vi "Find Relay Index.vi"(8 "error in (no error)":errorcluster, 10 "relay string":string, 11 "SLSC Switch in":refnum<class "SLSC Switch.lvclass">) -> (0 "error out":errorcluster, 2 "index":i32, 3 "SLSC Switch out":refnum<class "SLSC Switch.lvclass">)   [LabVIEW 2016, in "SLSC Switch.lvlib" / "SLSC Switch.lvclass"]
uses:
  SLSC Switch.lvclass
  SLSC Switch.lvclass/SLSC Switch.ctl
  Switch Action Processor/Switch Action Processor.lvclass/Switch Action Processor.ctl
  Relay/Relay.lvclass/Relay.ctl
  Relay/Relay.lvclass
  Switch Action Processor/Switch Action Processor.lvclass
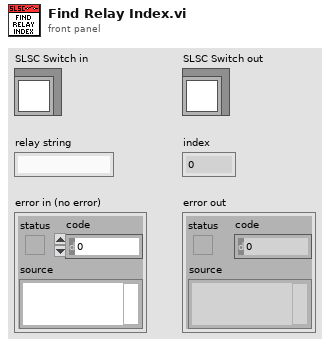
[diagram p1: front panel]
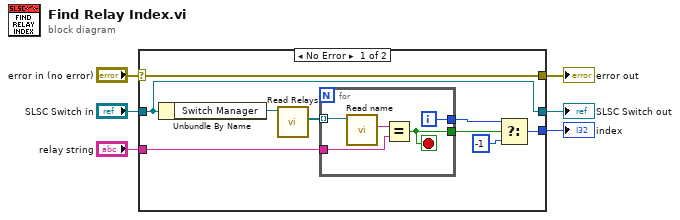
[diagram p0: block diagram]
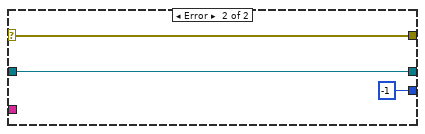
[diagram p2: hidden frame]
diagram:
  n1 = case shown="No Error" "error in (no error)" {
    selector: "error in (no error)" -> [w13 w23]
    tunnel: [w13 w23] -> w5
    tunnel: "relay string" -> [w15 _]
    tunnel: [w14 -1 ("index of element")] -> w3
    tunnel: "SLSC Switch in" -> [w9 w21]
    tunnel: [w9 w21] -> w1
    frame No Error {
      n2 = Unbundle By Name(w9) -> ("Switch Manager"=w8:refnum<class "Switch Action Processor.lvclass">)
      n3 = call "Read Relays.vi"("Switch Action Processor in"=w8) -> ("Relays"=w7:refnum<class "Relay.lvclass">[])  [unwired: 9 in, 1 out]
      n4 = for {
        tunnel: w7 -> [w17] mode=indexing
        tunnel: w15 -> [w20]
        tunnel: [w19] -> w11
        tunnel: [w18] -> w12
        i -> [w19]
        stop <- w18 stop-if-true
        n5 = call "Read name.vi"("Relay in"=w17) -> ("name"=w16:string)  [unwired: 8 in, 2 out]
        n6 = Equal?(x=w16, y=w20) -> (x = y?=w18:bool)
      }
      n7 = Select(t=w11, s=w12, f=-1) -> (s? t:f=w14:i32)
    }
    frame Error {
    }
  }
  "error out" <- w5
  "index" <- w3
  "SLSC Switch out" <- w1
